vi "Front Switch.vi"(8 "Command Info In":T2, 10 "Block Inputs":T1, 11 "Starting Position":T5=enum."Far Right") -> (0 "Command Info Out":T2)   [LabVIEW 2017]
uses:
  Support Code/Starting Position.ctl
  <vilib>/Rock Robotics/WPI/Framework/Command Status Info.ctl
  <vilib>/Rock Robotics/WPI/Framework/Completion Status.ctl
  <vilib>/Rock Robotics/WPI/Framework/Completion Notifier.ctl
  Block Clusters/Front Switch.ctl
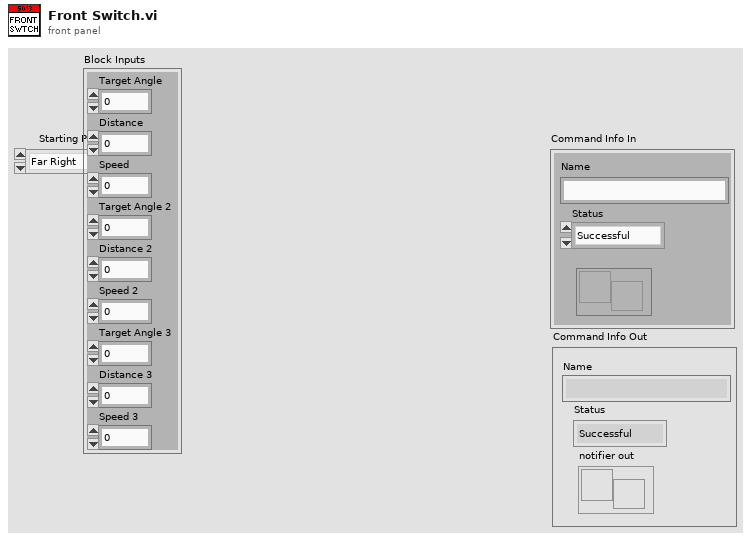
[diagram p1: front panel]
types:
  T1 = typedef "Front Switch.ctl" = cluster{"Target Angle":dbl, "Distance":dbl, "Speed":dbl, "Target Angle 2":dbl, "Distance 2":dbl, "Speed 2":dbl, "Target Angle 3":dbl, "Distance 3":dbl, "Speed 3":dbl}
  T2 = typedef "Command Status Info.ctl" = cluster{"Name":string, "Status":T3, "notifier out":T4}
  T3 = typedef "Completion Status.ctl" = enum16{"Successful", "Aborted", "Incomplete"}
  T4 = typedef "Completion Notifier.ctl" = refnum<notifier>
  T5 = typedef "Starting Position.ctl" = enum16{"Far Left", "Center", "Far Right"}
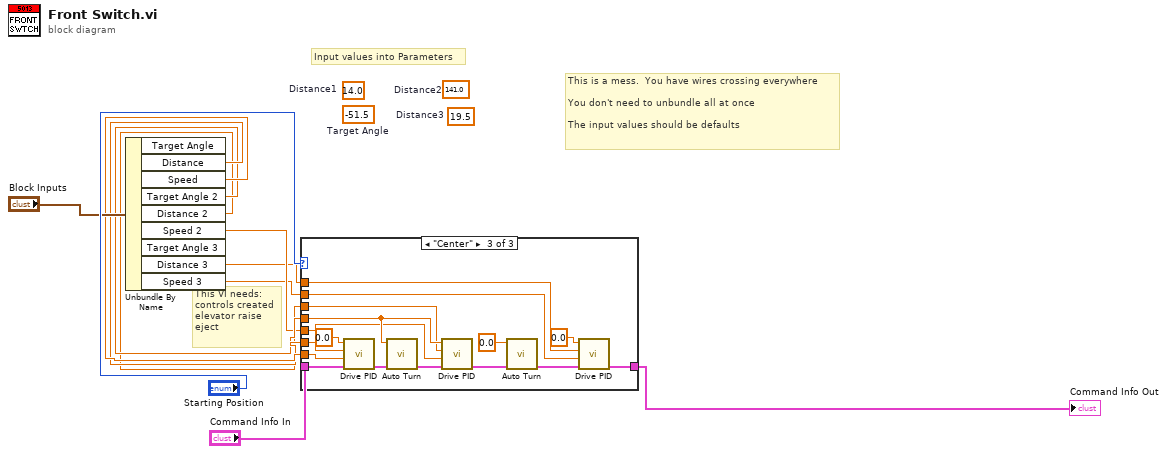
[diagram p0: block diagram]
diagram:
  (unwired) 19.5  # Distance3
  (unwired) 141.0  # Distance2
  (unwired) -51.5  # Target Angle
  (unwired) 14.0  # Distance1
  # "This is a mess.  You have wires crossing everywhere\n\nYou don't need to unbundle all at once\n\nThe input values should be defaults"
  # "Input values into Parameters"
  # "This VI needs:\ncontrols created\nelevator raise\neject"
  n1 = Unbundle By Name("Block Inputs") -> ("Distance"=w6:dbl, "Speed"=w8:dbl, "Target Angle 2"=w5:dbl, "Distance 2"=w4:dbl, "Speed 2"=w3:dbl, "Distance 3"=w2:dbl, "Speed 3"=w1:dbl)  [unwired: 2 out]
  n2 = case shown="\"Center\"" "Starting Position" {
    tunnel: "Command Info In" -> [w12 w13 w23]
    tunnel: w8 -> [_ _ w22]
    tunnel: [w12 w13 w20] -> w7
    tunnel: w6 -> [_ _ w19]
    tunnel: w5 -> [_ _ w18]
    tunnel: w4 -> [_ _ w17]
    tunnel: w3 -> [_ _ w16]
    tunnel: w2 -> [_ _ w15]
    tunnel: w1 -> [_ _ w14]
    frame "Far Left" {
    }
    frame "Far Right", Default {
    }
    frame "Center" {
      n3 = call "Drive PID.vi"("Command Info In"=w23, "Speed"=w22, "Distance"=w19, "Target Angle"=0.0) -> ("Command Info Out"=w29:T2)  [unwired: 7 in]
      n4 = call "Auto Turn.vi"("Command Info In"=w29, "Target Angle"=w18) -> ("Command Info Out"=w28:T2)  [unwired: 9 in]
      n5 = call "Drive PID.vi"("Command Info In"=w28, "Speed"=w16, "Distance"=w17, "Target Angle"=w18) -> ("Command Info Out"=w27:T2)  [unwired: 7 in]
      n6 = call "Auto Turn.vi"("Command Info In"=w27, "Target Angle"=0.0) -> ("Command Info Out"=w26:T2)  [unwired: 9 in]
      n7 = call "Drive PID.vi"("Command Info In"=w26, "Speed"=w14, "Distance"=w15, "Target Angle"=0.0) -> ("Command Info Out"=w20:T2)  [unwired: 7 in]
    }
  }
  "Command Info Out" <- w7
